vi "Display Images New.vi"(0 "fpga interface in":refnum<k20>, 1 "'stop' notifier":refnum<notifier>, 5 "display channel number":i32, 7 "raw display notifier":refnum<notifier>, 11 "error in (no error)":errorcluster) -> (4 "fpga interface out":refnum<k20>, 15 "error out":errorcluster)   [LabVIEW 2026]
uses:
  Types/Serial Channel Display Parameters.ctl
  <vilib>/vision/Image Controls.llb/IMAQ Image.ctl
  Types/RAW Interpretation for Display.ctl
  FPGA/Common/Types/Image Metadata.ctl
  <instrlib>/FlexRIO/CSI-2/v2/Common/Types/LLP Data Type.ctl
  Types/148x_Common_FPGA_Reference.ctl
  <vilib>/Utility/error.llb/Error Cluster From Error Code.vi
  <vilib>/rvi/errors/niLvFpgaAdjustHostInterfaceError.vi
  <vilib>/rvi/interface/nirviReadWriteControl/nirviReadWriteControl.xnode
  GettingStarted_Common_148X_Host.lvlib
  NiFpgaLv.dll
  <vilib>/rvi/interface/Simulation/niFpgaSimulationCallBeginRW.vi
  <instrlib>/FlexRIO/CSI-2/v2/Common/NI CSI-2 API Common v2.lvlib
  FPGA/Common/GettingStarted_Common_148X_FPGA.lvlib
panel:
  out "size(s)":i32
  out "image metadata":T1[](array[typedef])
  out "Acquired Frames/s":dbl
  out "Processed Frames/s":dbl
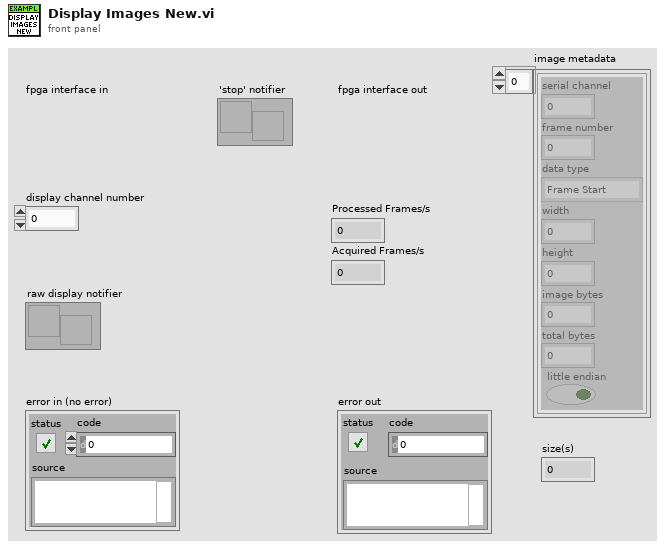
[diagram p1: front panel]
types:
  T1 = typedef "GettingStarted_Common_148X_FPGA.lvlib/Image Metadata.ctl" = cluster{"serial channel":fxp<+,3,3>, "frame number":u16, "data type":T2, "width":u16, "height":u16, "image bytes":u32, "total bytes":u32, "little endian":bool}
  T2 = typedef "NI CSI-2 API Common v2.lvlib/LLP Data Type.ctl" = enum8{"Frame Start", "Frame End", "Line Start", "Line End", "End of Transmission", "Reserved 0", "Reserved 1", "Reserved 2", "Generic Short Packet 1", "Generic Short Packet 2", "Generic Short Packet 3", "Generic Short Packet 4", "Generic Short Packet 5", "Generic Short Packet 6", "Generic Short Packet 7", "Generic Short Packet 8", "Null", "Blanking Data", "Embedded 8-bit non Image Data", "Generic Long Packet 1", "Generic Long Packet 2", "Generic Long Packet 3", "Generic Long Packet 4", "Reserved 3", "YUV420 8-bit", "YUV420 10-bit", "Legacy YUV420 8-bit", "Reserved 4", "YUV420 8-bit Chroma Shifted", "YUV420 10-bit Chroma Shifted", "YUV422 8-bit", "YUV422 10-bit", "RGB444", "RGB555", "RGB565", "RGB666", "RGB888", "Reserved 5", "Reserved 6", "RAW 24", "RAW 6", "RAW 7", "RAW 8", "RAW 10", "RAW 12", "RAW 14", "RAW 16", "RAW 20", "User Defined 8-bit Data 1", "User Defined 8-bit Data 2", "User Defined 8-bit Data 3", "User Defined 8-bit Data 4", "User Defined 8-bit Data 5", "User Defined 8-bit Data 6", "User Defined 8-bit Data 7", "User Defined 8-bit Data 8", "USL Command", "Reserved 7", "Reserved 8", "Reserved 9", "Reserved 10", "Reserved 11", "Reserved 12", "LRTE EPD Spacer"}
  T3 = typedef "GettingStarted_Common_148X_Host.lvlib/148x_Common_FPGA_Reference.ctl" = refnum<k20>
  T4 = typedef "GettingStarted_Common_148X_Host.lvlib/Serial Channel Display Parameters.ctl" = cluster{"images":cluster{"grayscale":T5, "color":T5}, "RAW parameters":cluster{"interpretation":T6, "bayer parameters":cluster{"pattern":i32, "algorithm":i32, "red gain":dbl, "green gain":dbl, "blue gain":dbl}}}
  T5 = typedef "IMAQ Image.ctl" = refnum<image>
  T6 = typedef "GettingStarted_Common_148X_Host.lvlib/RAW Interpretation for Display.ctl" = enum16{"Grayscale", "Bayer", "RGB", "YUV422", "YUV420", "Legacy YUV420"}
  T7 = cluster{"image pixel data fifo overflow":bool, "image metadata fifo overflow":bool}[]
  T8 = cluster{"image pixel data fifo overflow":bool, "image metadata fifo overflow":bool}
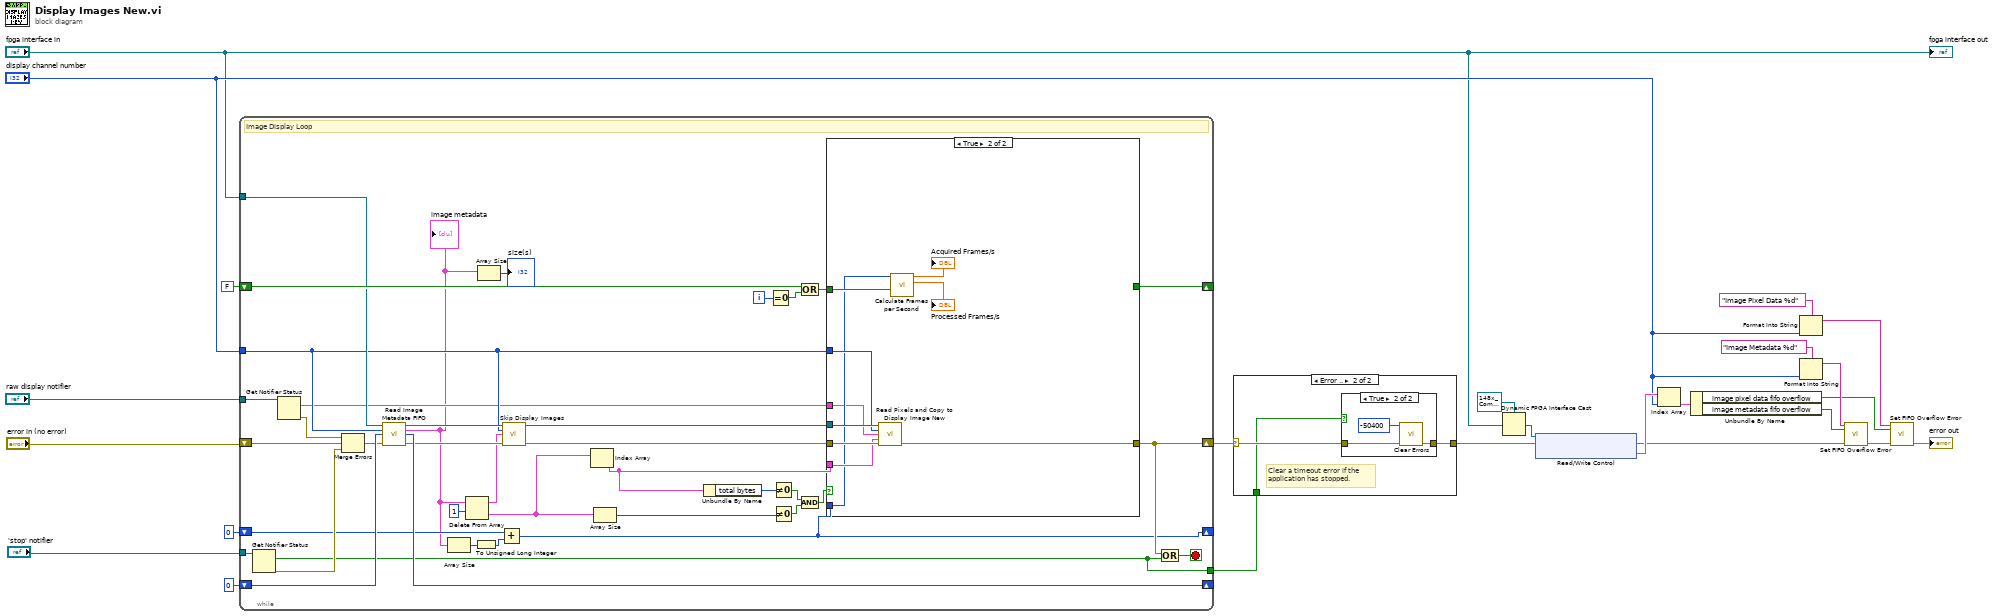
[diagram p0: block diagram]
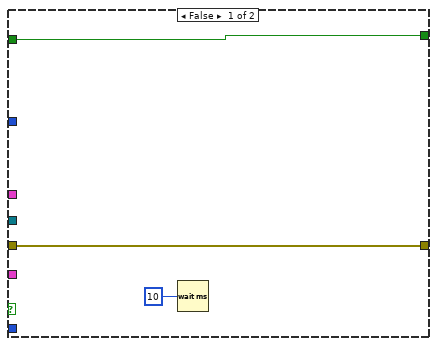
[diagram p2: hidden frame]
diagram:
  n1 = while {
    shift-right: [w59] -> w6
    shift-left: "error in (no error)" -> [w31]
    tunnel: "fpga interface in" -> [w35]
    shift-right: [w60] -> _
    shift-left: u32 0 ("Elements Remaining") -> [w48]
    tunnel: "display channel number" -> [w30]
    shift-right: [w52] -> _
    shift-left: FALSE -> [w49]
    shift-right: [w36] -> _
    shift-left: u32 0 ("Elements Remaining") -> [w39]
    tunnel: [w33] -> w3
    tunnel: "'stop' notifier" -> [w34]
    tunnel: "raw display notifier" -> [w29]
    i -> [w58]
    stop <- w61 stop-if-true
    # "Image Display Loop"
    n2 = Get Notifier Status(notifier=w34) -> (current notification=w33:bool, error out=w62:errorcluster)  [unwired: 1 in, 3 out]
    n3 = Get Notifier Status(notifier=w29) -> (current notification=w28:T4[], error out=w27:errorcluster)  [unwired: 1 in, 3 out]
    n4 = Merge Errors(w27, w31, w62) -> (w32:errorcluster)
    n5 = call "Read Image Metadata FIFO.vi"("fpga inteface in"=w35, "display channel number"=w30, "number of images"=w48, "error in (no error)"=w32) -> ("fpga interface out"=w44:refnum<k20>, "image metadata"=w26:T1[], "images remaining"=w60:u32, "error out"=w41:errorcluster)  [unwired: 8 in]
    "image metadata" <- w26
    n6 = Array Size(array=w26) -> (size(s)=w38:i32)
    n7 = Delete From Array(array=w26, length=1) -> (deleted portion=w45:T1[], array with subset deleted=w40:T1[])  [unwired: 1 in]
    n8 = To Unsigned Long Integer(number=w38) -> (unsigned 32bit integer=w37:u32)
    n9 = Array Size(array=w26) -> (size(s)=→"size(s)":i32)
    n10 = Add(x=w39, y=w37) -> (x+y=w36:u32)
    n11 = call "Skip Display Images.vi"("fpga interface in"=w44, "display channel number"=w30, "image metadata"=w40, "error in (no error)"=w41) -> ("fpga interface out"=w43:refnum<k20>, "error out"=w42:errorcluster)  [unwired: 10 in]
    n12 = Index Array(array=w45) -> (element=w57:T1)  [unwired: 1 in]
    n13 = Array Size(array=w45) -> (size(s)=w47:i32)
    n14 = Unbundle By Name(w57) -> ("total bytes"=w56:u32)
    n15 = Equal To 0?(x=w58) -> (x = 0?=w50:bool)
    n16 = Not Equal To 0?(x=w56) -> (x != 0?=w54:bool)
    n17 = Not Equal To 0?(x=w47) -> (x != 0?=w55:bool)
    n18 = Compound Arithmetic op=OR(w49, w50) -> (w51:bool)
    n19 = Compound Arithmetic op=AND(w54, w55) -> (w53:bool)
    n20 = case shown="True" w53 {
      tunnel: w42 -> [w65 w75]
      tunnel: w43 -> [_ w74]
      tunnel: w28 -> [_ w68]
      tunnel: w30 -> [_ w73]
      tunnel: [w65 w69] -> w59
      tunnel: w57 -> [_ w72]
      tunnel: w51 -> [w63 w71]
      tunnel: [w63 _] -> w52
      tunnel: w36 -> [_ w70]
      frame False {
        n21 = Wait (ms)(milliseconds to wait=u32 10) -> ()  [unwired: 1 out]
      }
      frame True {
        n22 = call "Read Pixels and Copy to Display Image New.vi"("fpga interface in"=w74, "display channel number"=w73, "serial channel display parameters"=w68, "image metadata"=w72, "error in (no error)"=w75) -> ("error out"=w69:errorcluster)  [unwired: 7 in, 3 out]
        n23 = call <vilib>:"Calculate Frames per Second.vi"("Reset"=w71, "Buffer Number"=w70) -> ("Processed Frames/s"=→"Processed Frames/s":dbl, "Acquired Frames/s"=→"Acquired Frames/s":dbl)  [unwired: 7 in, 1 out]
      }
    }
    n24 = Compound Arithmetic op=OR(w59, w33) -> (w61:bool)
  }
  n25 = case shown="Error .." w6 {
    selector: w6 -> [w76 w79]
    tunnel: [w76 w78] -> w19
    tunnel: w3 -> [_ w77]
    frame No Error {
    }
    frame Error {
      # "Clear a timeout error if the application has stopped."
      n26 = case shown="True" w77 {
        tunnel: w79 -> [w80 w83]
        tunnel: [w80 w81] -> w78
        frame False {
        }
        frame True {
          n27 = call <vilib>:"Clear Errors.vi"("error in (no error)"=w83, "specific error code to clear (0: all)"=-50400 ("y")) -> ("error out"=w81:errorcluster)  [unwired: 4 in, 1 out]
        }
      }
    }
  }
  n28 = Dynamic FPGA Interface Cast(Session In=T3 refnum ("FPGA VI Reference Out"), Type="fpga interface in") -> (Session Out=w20:T3)
  n29 = xnode "Read/Write Control"("FPGA VI Reference In"=w20, "error in"=w19) -> ("error out"=w18:errorcluster, "display channel status"=w22:T7)  [unwired: 1 out]
  n30 = Index Array(array=w22, index="display channel number") -> (element=w23:T8)
  n31 = Unbundle By Name(w23) -> ("image pixel data fifo overflow"=w10:bool, "image metadata fifo overflow"=w9:bool)
  n32 = Format Into String(format string="Image Pixel Data %d", "display channel number") -> (resulting string=w12:string)  [unwired: 2 in, 1 out]
  n33 = Format Into String(format string="Image Metadata %d", "display channel number") -> (resulting string=w11:string)  [unwired: 2 in, 1 out]
  n34 = call "Set FIFO Overflow Error.vi"("fifo name"=w11, "overflow"=w9, "error in (no error)"=w18) -> ("error out"=w14:errorcluster)  [unwired: 12 in]
  n35 = call "Set FIFO Overflow Error.vi"("fifo name"=w12, "overflow"=w10, "error in (no error)"=w14) -> ("error out"=→"error out":errorcluster)  [unwired: 12 in]
  "fpga interface out" <- "fpga interface in"
